vi "PH_Beamline_Chief.ProcCases.vi"(0 "i ref in":refnum<vi>, 1 "selector":string, 2 "Data":T1, 3 "call cluster":T2={"Object"="", "Selector"="", "CallType"=enum."synchronous", "Async Object"="", "Async Selector"="", "Data Descriptor"="", "Data"=[], "Error #"=0, "Expire"=0}, 5 "error in (no error)":errorcluster) -> (14 "i ref out":refnum<vi>, 17 "answer cluster":T2={"Object"="", "Selector"="", "CallType"=enum."synchronous", "Async Object"="", "Async Selector"="", "Data Descriptor"="", "Data"=[], "Error #"=0, "Expire"=0}, 19 "error out":errorcluster)   [LabVIEW 2014, in "PH_Beamline_Chief.lvlib"]
doc: "This method is called by a process from within the default case in the event loop. The methods of a class that are linked to events will be called from THIS method. Add your code here."
uses:
  PH_Beamline_Chief.lvlib
  CS_Core/CSSystem/CoreDefs/CoreDefs.call_type.ctl
  CS_Core/BaseProcess/BaseProcess.descriptor string definition.ctl
  CS_Core/CSSystem/CoreDefs/CoreDefs.rawDataType.ctl
  PH_Beamline_Chief.Settings.ctl
  CS_Core/CSSystem/CoreLib/CoreLib.byte array 2 short.vi
  CS_Core/CSSystem/CoreLib/CoreLib.string 2 byte array.vi
  PH_Beamline/PH_Beamline.lvlib
  PH_BL-Master/PH_BL-Master.lvlib
  PH_Basics/PH_SystemInformation/PH_SystemInformation.lvlib
  CS_Core/CSSystem/CoreLib/CoreLib.lvlib
  CS_Core/BaseProcess/BaseProcess.lvlib
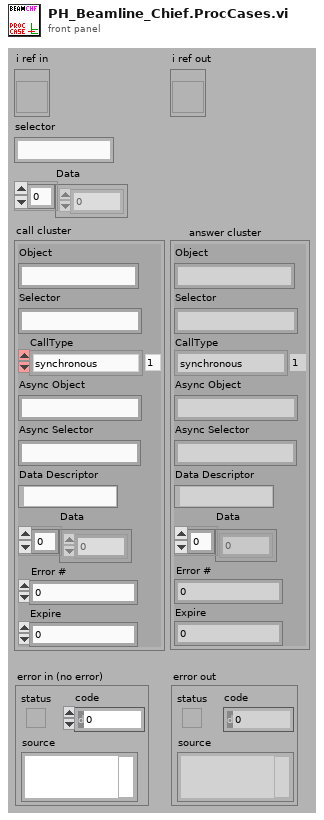
[diagram p1: front panel]
types:
  T1 = typedef "CoreDefs.rawDataType.ctl" = i8[]
  T2 = typedef "CoreDefs.call_type.ctl" = cluster{"Object":string, "Selector":string, "CallType":enum16{"simple", "synchronous", "asynchronous"}, "Async Object":string, "Async Selector":string, "Data Descriptor":T3, "Data":T1, "Error #":i32, "Expire":u32}
  T3 = typedef "BaseProcess.lvlib/BaseProcess.descriptor string definition.ctl" = string
  T4 = enum16{"Laser", "PreAmp", "MainAmp", "Exp 1", "Exp 2", "Exp 3", "Exp 4"}
  T5 = typedef "PH_Beamline_Chief.lvlib/PH_Beamline_Chief.Settings.ctl" = cluster{"PA Doublepass Mode":bool, "Compressor Vaccuum LB not relevant":bool, "Windowshutter TB2 not relevant":bool, "Windowshutter TB3 not relevant":bool}
  T6 = typedef "PH_BL-Master.lvlib/PH_BL-Master.i attribute.ctl" = cluster{"Remote controlled":bool, "Boolean Condition Service Subscriber":refnum<vi>[], "Picture Condition Service Subscriber":refnum<vi>[], "R2S":cluster{"GUI Ref":refnum<vi>, "State":bool}, "Vacua":cluster{"GUI Ref":refnum<vi>, "Limit":dbl, "Curr Value":dbl, "in range":bool}[], "O2 Inspection":cluster{"GUI Ref":refnum<vi>, "Concentration":dbl, "State":T7}[], "Boolean Status Service Subscriber":cluster{"GUI Ref":refnum<vi>, "Status":T7, "no Link?":bool, "Status Subscriber Class":T8}[], "Picture Status Service Subscriber":cluster{"GUI Ref":refnum<vi>, "Status":T7, "no Link?":bool, "Status Subscriber Class":T8}[], "6P 4Q Service Subscriber":cluster{"GUI Ref":refnum<vi>, "Selector":T9, "no Link?":bool}[], "Index of latest 6P 4Q changing Instance":i32, "Index of latest Picture Status changing Instance":i32, "Index of latest Boolean Status changing Instance":i32, "Vision ID on same Node":string, "Start Phase over?":bool, "GUI Ref Delete":refnum<vi>}
  T7 = typedef "PH_StatusHandler.lvlib/PH_StatusHandler.Status.ctl" = i16
  T8 = typedef "PH_BL-Master.lvlib/PH_BL-Master.Status Subscriber Class.ctl" = enum16{"unknown", "Switch", "BB", "6P Switch", "Switch GUI", "Switch and 6P State", "Force Sensor"}
  T9 = typedef "PH_4_Pos_Selector.lvlib/PH_4_Pos_Selector.Position Selector.ctl" = u16
  T10 = cluster{"GUI Ref":refnum<vi>, "Status":T7, "no Link?":bool, "Status Subscriber Class":T8}[]
  T11 = cluster{"GUI Ref":refnum<vi>, "Limit":dbl, "Curr Value":dbl, "in range":bool}[]
  T12 = typedef "PH_Beamline.lvlib/PH_Beamline.i attribute.ctl" = cluster{"GUI Refs":cluster{"PA ok":refnum<vi>, "MA ok":refnum<vi>, "fs FE ok":refnum<vi>, "ns FE ok":refnum<vi>, "PA ED ok":refnum<vi>, "MAS ok":refnum<vi>, "Booster ok":refnum<vi>, "Mirrortower ok":refnum<vi>, "In.-Box ok":refnum<vi>, "Compressor ok":refnum<vi>, "Experiment LB ok":refnum<vi>, "Experiment LL ok":refnum<vi>, "PHELIX_Beckhoff_Watchdog":refnum<vi>, "Shutters closed":refnum<vi>, "uOPA ok":refnum<vi>, "Vacuum no shotcond Comp LB":refnum<vi>}, "Refs BL MA":refnum<vi>[], "Refs BL MA-IB":refnum<vi>[], "Refs BL fs":refnum<vi>[], "Refs BL PA ED":refnum<vi>[], "Refs BL MAS":refnum<vi>[], "Refs BL Boo":refnum<vi>[], "Refs BL ns":refnum<vi>[], "Refs BL Mirrortower":refnum<vi>[], "Refs BL Compressor":refnum<vi>[], "Refs BL Exp LB":refnum<vi>[], "Radiation Safety":cluster{"Exp Laserbay":cluster{"Ref Op Mode":refnum<vi>, "Ref Laserbay evacuated":refnum<vi>, "Tagname LB evacuated":string, "Shot Mode":T13, "Laserbay evacuated?":i32, "Tagname HV room locked":string, "HV room locked?":i32, "Ref HV room locked":refnum<vi>, "Tagname bridged?":string, "Ref Bridge":refnum<vi>, "I<1E18W/cm²":bool}, "Exp Laserlab":cluster{"Ref Op Mode":refnum<vi>, "Ref Laserlab evacuated":refnum<vi>, "Tagname LL evacuated":string, "Shot Mode":T13, "Laserlab evacuated?":i32, "Tagname bridged?":string, "Ref Bridge":refnum<vi>, "I<1E18W/cm²":bool}}, "Refs BL LL":refnum<vi>[], "PP Igni Heating GUI Refs":refnum<vi>[], "PP Igni Heating Tagnames ":string[], "Refs BL PA":cluster{"undelayed Line before Shutter":refnum<vi>[], "undelayed Line after Shutter":refnum<vi>[], "before Bypass":refnum<vi>[], "delayed Line before Shutter":refnum<vi>[], "delayed Line after Shutter":refnum<vi>[], "before Shutter Input":refnum<vi>[], "after Shutter Input":refnum<vi>[], "Bypass":refnum<vi>[], "before Shutter Exit":refnum<vi>[], "after Shutter Exit":refnum<vi>[], "to MA":refnum<vi>[], "to Lab":refnum<vi>[]}, "BL":cluster{"YLF_BL_Status":i32, "fs_BL_Status":i32, "fs_YLF_BL_Status":i32, "ns_BL_Status":i32, "PA_Input_BL_Status":i32, "PA_UnDelay_BL_Status":i32, "PA_Delay_BL_Status":i32, "PA_BL_Status":i32, "PA_Bypass_BL_Status":i32, "PA_Exit_BL_Status":i32, "PA_LL_BL_Status":i32, "LL_BL_Status":i32, "PA_MA_BL_Status":i32, "MA_Exit_BL_Status":i32, "MA_Z6_BL_Status":i32, "Z6_BL_Status":i32, "MA_LB_BL_Status":i32, "LB_TB2_BL_Status":i32, "PA_before_Bypass_BL_Status":i32, "LB_TB3_BL_Status":i32}, "State Subsystems":cluster{"PA":bool, "MA":bool, "ns FE":bool, "fs FE":bool, "PA ED":bool, "In.-Box":bool, "MAS":bool, "Booster":bool, "Mirrortower":bool, "Compressor":bool, "Experiment LB":bool, "Experiment LL":bool, "uOPA":bool}, "Status Subscriber Information":T14, "Refs BL uOPA":refnum<vi>[], "PA_Input_2_Beam_6PWpGUI not linked?":bool, "PA_Input_Delay_6PGUI not linked?":bool, "Settings":T5}
  T13 = typedef "PH_Beamline.lvlib/PH_Beamline.Operation Mode.ctl" = i32
  T14 = typedef "PH_Beamline.lvlib/PH_Beamline.Status Subscriber Information.ctl" = cluster{"fs Swich YLF":T15, "fs Exit Shutter":T15, "ns Exit Shutter":T15, "PA Input Shutter":T15, "PA PC WP":T15, "PA PC WP 2":T15, "PA Bypass In":T15, "PA Bypass Out":T15, "PA CH 1":T15, "PA delayed":T15, "PA non delayed":T15, "PA Exit Shutter":T15, "PA Switch Lab":T15, "PA Bridge CH Input MA":T15, "MA Diffusor IB":T15, "MA IB Ready":T15, "MA CH 1":T15, "MA CH 2":T15, "MA CH 3":T15, "MA CH 4":T15, "MA Shutter Align Cam":T15, "MA Position MM5":T15, "Calorimeter Switch":T15, "BL Z6 CH 9":T15, "BL Z6 Beamdump":T15, "BL Z6 Shutter":T15, "COS Sensitivity Switch":T15, "Exp LB Shutter":T15, "Exp LB TB 2":T15, "Exp LB TB 3":T15, "PA LL Input CH":T15, "PA LL Output CH":T15, "LL Comp Input Shutter":T15, "LL Comp Output Shutter":T15, "LL Comp FF Shutter":T15, "Exp LL Shutter":T15, "MA IM In IB":T15, "MA IM Out IB":T15, "MA DB In IB":T15, "MA DB Out IB":T15, "Exp LB Shutter Interlock":T15, "Exp LL Shutter Interlock":T15, "MM1 Force Sensor":T15}
  T15 = typedef "PH_BL-Master.lvlib/PH_BL-Master.Status Subscriber Information.ctl" = cluster{"Index of element":i32, "Attributeset":T16}
  T16 = typedef "PH_BL-Master.lvlib/PH_BL-Master.Attribute Set.ctl" = enum16{"Boolean Status Service Subscriber", "Picture Status Service Subscriber"}
  T17 = cluster{"YLF_BL_Status":i32, "fs_BL_Status":i32, "fs_YLF_BL_Status":i32, "ns_BL_Status":i32, "PA_Input_BL_Status":i32, "PA_UnDelay_BL_Status":i32, "PA_Delay_BL_Status":i32, "PA_BL_Status":i32, "PA_Bypass_BL_Status":i32, "PA_Exit_BL_Status":i32, "PA_LL_BL_Status":i32, "LL_BL_Status":i32, "PA_MA_BL_Status":i32, "MA_Exit_BL_Status":i32, "MA_Z6_BL_Status":i32, "Z6_BL_Status":i32, "MA_LB_BL_Status":i32, "LB_TB2_BL_Status":i32, "PA_before_Bypass_BL_Status":i32, "LB_TB3_BL_Status":i32}
  T18 = typedef "PH_SystemInformation.lvlib/PH_SystemInformationEnabling State.ctl" = i32
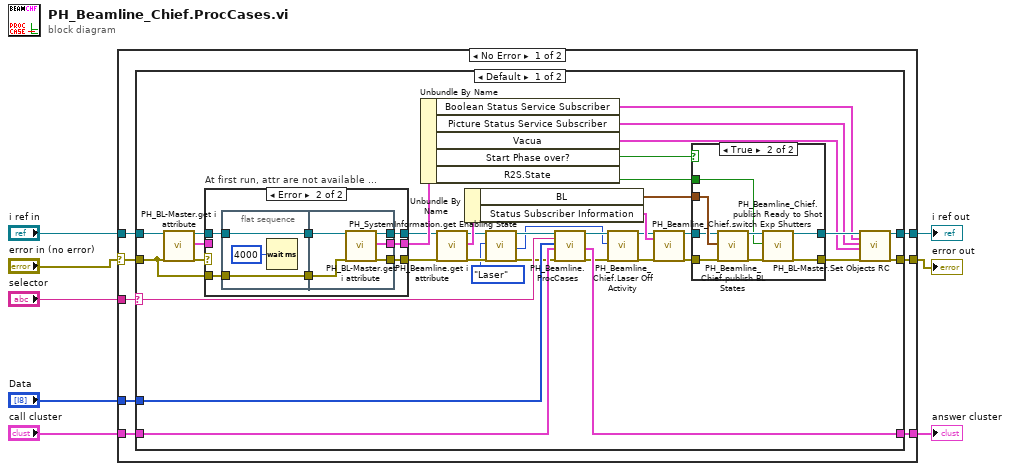
[diagram p0: block diagram]
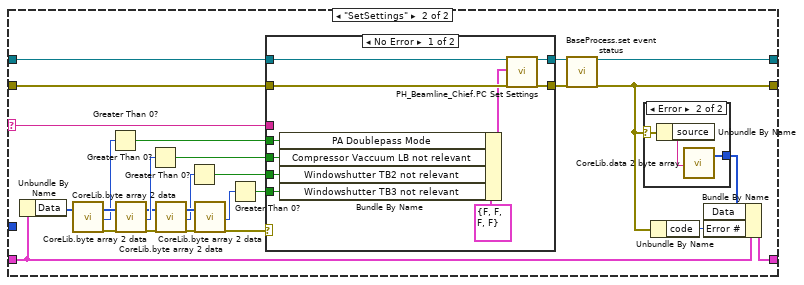
[diagram p4: hidden frame]
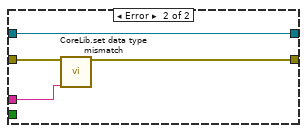
[diagram p5: hidden frame]
diagram:
  n1 = case shown="No Error" "error in (no error)" {
    selector: "error in (no error)" -> [w9 w126]
    tunnel: "selector" -> [w16 _]
    tunnel: [w15 w125] -> w7
    tunnel: "call cluster" -> [w14 w125]
    tunnel: "i ref in" -> [w13 w127]
    tunnel: [w12 w127] -> w4
    tunnel: [w11 w126] -> w3
    tunnel: "Data" -> [w10 _]
    frame No Error {
      n2 = case shown="Default" w16 {
        selector: w16 -> [w50 w81]
        tunnel: w13 -> [w20 w92]
        tunnel: [w43 w87] -> w12
        tunnel: w14 -> [w51 w85]
        tunnel: [w52 w86] -> w15
        tunnel: w9 -> [w23 w91]
        tunnel: [w45 w84] -> w11
        tunnel: w10 -> [w49 _]
        frame Default {
          n3 = call "PH_BL-Master.get i attribute.vi"("i ref in"=w20, "error in (no error)"=w23) -> ("i ref out"=w19:refnum<vi>, "i attribute"=w21:T6, "error out"=w22:errorcluster)  [unwired: 15 in]
          n4 = case "At first run, attr are not available ..." shown="Error" w22 {
            selector: w22 -> [w55 _]
            tunnel: [w55 w62] -> w47
            tunnel: w19 -> [w53 w61]
            tunnel: [w54 w60] -> w46
            tunnel: [w53 w59] -> w36
            tunnel: w23 -> [_ w58]
            tunnel: w21 -> [w54 _]
            frame No Error {
            }
            frame Error {
              n5 = flat-sequence {
                tunnel: w58 -> [w64]
                tunnel: w61 -> [w65]
                tunnel: [w65] -> w57
                tunnel: [w64] -> w56
                tunnel: [w70] -> w62
                tunnel: [w68] -> w60
                tunnel: [w67] -> w59
                tunnel: w57 -> [w69]
                tunnel: w56 -> [w66]
                frame #0 {
                  n6 = Wait (ms)(milliseconds to wait=u32 4000) -> ()  [unwired: 1 out]
                }
                frame #1 {
                  n7 = call "PH_BL-Master.get i attribute.vi"("i ref in"=w69, "error in (no error)"=w66) -> ("i ref out"=w67:refnum<vi>, "i attribute"=w68:T6, "error out"=w70:errorcluster)  [unwired: 15 in]
                }
              }
            }
          }
          n8 = Unbundle By Name(w46) -> ("Boolean Status Service Subscriber"=w39:T10, "Picture Status Service Subscriber"=w40:T10, "Vacua"=w41:T11, "Start Phase over?"=w48:bool, "R2S.State"=w17:bool)
          n9 = call "PH_Beamline.get i attribute.vi"("i ref in"=w36, "error in (no error)"=w47) -> ("i ref out"=w33:refnum<vi>, "i attribute"=w35:T12, "error out"=w32:errorcluster)  [unwired: 15 in]
          n10 = Unbundle By Name(w35) -> ("BL"=w18:T17, "Status Subscriber Information"=w34:T14)
          n11 = call "PH_SystemInformation.get Enabling State.vi"("i ref in"=w33, "Wanted State"=T4."Laser", "error in (no error)"=w32) -> ("i ref out"=w31:refnum<vi>, "Enabling State"=w24:T18, "error out"=w30:errorcluster)  [unwired: 14 in]
          n12 = call "PH_Beamline.ProcCases.vi"("i ref in"=w31, "selector"=w50, "Data"=w49, "call cluster"=w51, "error in (no error)"=w30) -> ("i ref out"=w26:refnum<vi>, "answer cluster"=w52:T2, "error out"=w25:errorcluster)  [unwired: 12 in]
          n13 = call "PH_Beamline_Chief.Laser Off Activity.vi"("i ref in"=w26, "Laser Enabling State before"=w24, "error in"=w25) -> ("i ref out"=w29:refnum<vi>, "error out"=w28:errorcluster)  [unwired: 15 in]
          n14 = call "PH_Beamline_Chief.switch Exp Shutters.vi"("i ref in"=w29, "Status Subscriber Information before"=w34, "error in"=w28) -> ("i ref out"=w38:refnum<vi>, "error out"=w37:errorcluster)  [unwired: 15 in]
          n15 = case shown="True" w48 {
            tunnel: [w72 w75] -> w42
            tunnel: [w71 w74] -> w44
            tunnel: w37 -> [w71 w78]
            tunnel: w38 -> [w72 w79]
            tunnel: w18 -> [_ w80]
            tunnel: w17 -> [_ w73]
            frame False {
            }
            frame True {
              n16 = call "PH_Beamline_Chief.publish BL States.vi"("i ref in"=w79, "BL States before"=w80, "error in (no error)"=w78) -> ("i ref out"=w76:refnum<vi>, "error out"=w77:errorcluster)  [unwired: 15 in]
              n17 = call "PH_Beamline_Chief.publish Ready to Shot.vi"("i ref in"=w76, "R2S before"=w73, "error in (no error)"=w77) -> ("i ref out"=w75:refnum<vi>, "error out"=w74:errorcluster)  [unwired: 15 in]
            }
          }
          n18 = call "PH_BL-Master.Set Objects RC.vi"("VI in"=w42, "Boolean Status Service Subscriber before"=w39, "Picture Status Service Subscriber before"=w40, "Vacua before"=w41, "error in (no error)"=w44) -> ("VI out"=w43:refnum<vi>, "error out"=w45:errorcluster)  [unwired: 13 in]
        }
        frame "SetSettings" {
          n19 = Unbundle By Name(w85) -> ("Data"=w104:T1)
          n20 = call-poly "CoreLib.byte array 2 data.vi"("byteArray"=w104) -> ("byteArray out"=w106:T1, "i16"=w99:i16, "error out"=w107:errorcluster)  [unwired: 16 in]
          n21 = Greater Than 0?(x=w99) -> (x > 0?=w96:bool)
          n22 = call-poly "CoreLib.byte array 2 data.vi"("byteArray"=w106, "error in (no error)"=w107) -> ("byteArray out"=w100:T1, "i16"=w105:i16, "error out"=w101:errorcluster)  [unwired: 15 in]
          n23 = Greater Than 0?(x=w105) -> (x > 0?=w95:bool)
          n24 = call-poly "CoreLib.byte array 2 data.vi"("byteArray"=w100, "error in (no error)"=w101) -> ("byteArray out"=w102:T1, "i16"=w98:i16, "error out"=w103:errorcluster)  [unwired: 15 in]
          n25 = Greater Than 0?(x=w98) -> (x > 0?=w94:bool)
          n26 = call-poly "CoreLib.byte array 2 data.vi"("byteArray"=w102, "error in (no error)"=w103) -> ("i16"=w97:i16, "error out"=w82:errorcluster)  [unwired: 15 in, 1 out]
          n27 = Greater Than 0?(x=w97) -> (x > 0?=w93:bool)
          n28 = case shown="No Error" w82 {
            tunnel: w96 -> [w116 _]
            tunnel: w95 -> [w115 _]
            tunnel: w94 -> [w114 _]
            tunnel: w93 -> [w113 _]
            tunnel: w92 -> [w112 w121]
            tunnel: w91 -> [w111 w120]
            tunnel: [w110 w121] -> w90
            tunnel: [w109 w119] -> w83
            tunnel: w81 -> [_ w118]
            frame No Error {
              n29 = Bundle By Name(cluster=T5 {"PA Doublepass Mode"=FALSE, "Compressor Vaccuum LB not relevant"=FALSE, "Windowshutter TB2 not relevant"=FALSE, "Windowshutter TB3 not relevant"=FALSE} ("Settings"), "PA Doublepass Mode"=w116, "Compressor Vaccuum LB not relevant"=w115, "Windowshutter TB2 not relevant"=w114, "Windowshutter TB3 not relevant"=w113) -> (w108:T5)
              n30 = call "PH_Beamline_Chief.PC Set Settings.vi"("VI in"=w112, "Settings"=w108, "error in (no error)"=w111) -> ("VI out"=w110:refnum<vi>, "error out"=w109:errorcluster)  [unwired: 15 in]
            }
            frame Error {
              n31 = call "CoreLib.set data type mismatch.vi"("error in (no error)"=w120, "error source"=w118) -> ("error out"=w119:errorcluster)  [unwired: 17 in]
            }
          }
          n32 = call "BaseProcess.set event status.vi"("i ref in"=w90, "error in (no error)"=w83) -> ("i ref out"=w87:refnum<vi>, "error out"=w84:errorcluster)  [unwired: 15 in, 1 out]
          n33 = case shown="Error" w84 {
            selector: w84 -> [_ w124]
            tunnel: [_ w122] -> w88
            frame No Error {
            }
            frame Error {
              n34 = Unbundle By Name(w124) -> ("source"=w123:string)
              n35 = call-poly "CoreLib.data 2 byte array.vi"("string"=w123) -> ("byteArray out"=w122:T1)  [unwired: 18 in]
            }
          }
          n36 = Unbundle By Name(w84) -> ("code"=w89:i32)
          n37 = Bundle By Name(cluster=w85, "Data"=w88, "Error #"=w89) -> (w86:T2)
        }
      }
    }
    frame Error {
    }
  }
  "answer cluster" <- w7
  "i ref out" <- w4
  "error out" <- w3
